vi "Generate User Event.vi"(6 "User Event Priority":T2=enum."normal priority", 8 "Error In":errorcluster, 9 "Data":variant, 10 "Event Handler Message":T1, 11 "User Event Reference":T3) -> (0 "Error Out":errorcluster)   [LabVIEW 2023, in "QSM - Alarms.lvlib"]
doc: "This VI generates a user event with the specified priority for the Queued Message Handler template."
uses:
  QSM - Alarms.lvlib
  Controls/Event Handler Message.ctl
  Controls/User Event Type.ctl
  <vilib>/event_ctls.llb/usereventprio.ctl
  Controls/User Event Reference.ctl
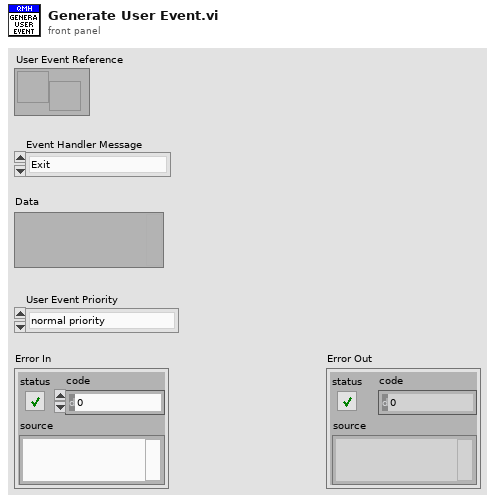
[diagram p1: front panel]
types:
  T1 = typedef "QSM - Alarms.lvlib/Event Handler Message.ctl" = enum16{"Exit"}
  T2 = typedef "usereventprio.ctl" = enum32{"high priority", "normal priority"}
  T3 = typedef "QSM - Alarms.lvlib/User Event Reference.ctl" = refnum<user-event>
  T4 = typedef "QSM - Alarms.lvlib/User Event Type.ctl" = cluster{"Event Handler Message":T1, "Data":variant}
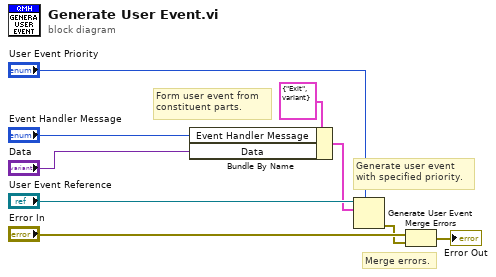
[diagram p0: block diagram]
diagram:
  # "Merge errors."
  # "Form user event from\nconstituent parts."
  # "Generate user event\nwith specified priority."
  n1 = Bundle By Name(cluster=T4 {"Event Handler Message"=enum."Exit", "Data"=variant} ("User Event Type"), "Event Handler Message"="Event Handler Message", "Data"="Data") -> (w6:T4)
  n2 = Generate User Event(priority (normal)="User Event Priority", user event="User Event Reference", event data cluster=w6) -> (error out=w1:errorcluster)  [unwired: 1 in, 1 out]
  n3 = Merge Errors("Error In", w1) -> (→"Error Out":errorcluster)
